vi "Play.vi"(8 "error in (no error)":errorcluster, 11 "Channel in":refnum<data-value>) -> (0 "error out":errorcluster, 3 "Channel out":refnum<data-value>)   [LabVIEW 2020, in "G-Audio.lvlib" / "Channel.lvclass"]
uses:
  Channel.lvclass
  Channel State.ctl
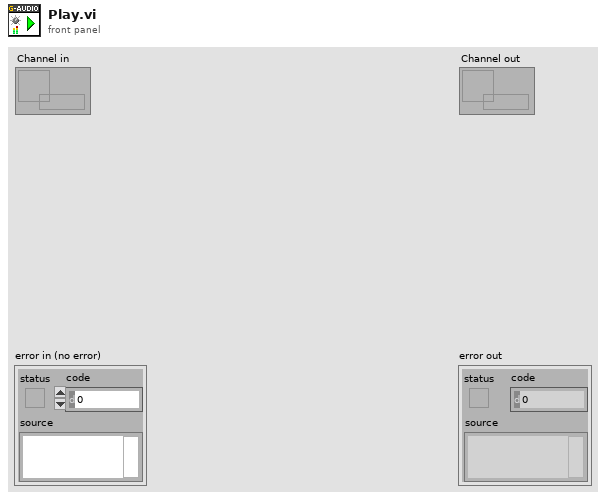
[diagram p1: front panel]
types:
  T1 = typedef "G-Audio.lvlib/Channel.lvclass/Channel State.ctl" = enum16{"Empty", "Loading", "Stopped", "Paused", "Playing", "Retrigger"}
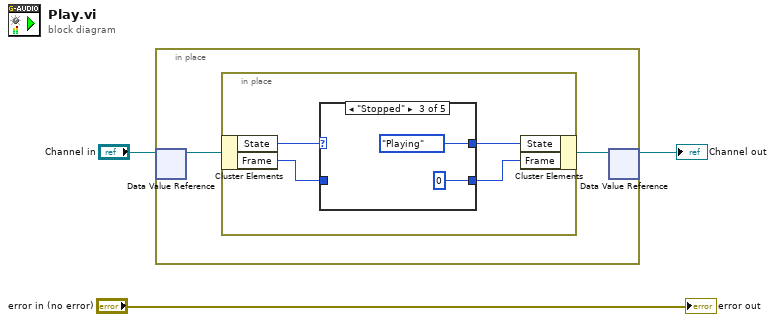
[diagram p0: block diagram]
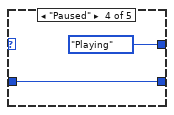
[diagram p4: hidden frame]
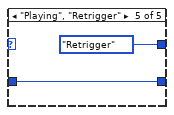
[diagram p5: hidden frame]
diagram:
  n1 = in-place {
    n2 = in-place-dvr #1("Channel in") -> (w5:refnum<class "Channel.lvclass">)  [unwired: 1 out]
    n3 = in-place {
      n4 = in-place-cluster #2(w5) -> ("State"=w9:T1, "Frame"=w7:u64)
      n5 = case shown="\"Stopped\"" w9 {
        selector: w9 -> [w11 w13 _ _ _]
        tunnel: [w11 w13 Channel_State."Playing" ("data value") Channel_State."Playing" ("data value") Channel_State."Retrigger" ("data value")] -> w8
        tunnel: [w10 w12 u64 0 ("Frame") w16 w18] -> w6
        tunnel: w7 -> [w10 w12 _ w16 w18]
        frame "Empty", Default {
        }
        frame "Loading" {
        }
        frame "Stopped" {
        }
        frame "Paused" {
        }
        frame "Playing", "Retrigger" {
        }
      }
      n6 = in-place-cluster #2("State"=w8, "Frame"=w6) -> (w4:refnum<class "Channel.lvclass">)
    }
    n7 = in-place-dvr #1(w4) -> (→"Channel out":refnum<data-value>)  [unwired: 1 out]
  }
  "error out" <- "error in (no error)"
